vi "Run Test - T90 Plot (SubVI).vi"(8 "error in (no error)":errorcluster, 11 "fileid":string) -> (0 "error out":errorcluster, 3 "Tengent Point":string)   [LabVIEW 2019]
uses:
  Controls/JSON - Report.ctl
  Controls/JSON - GetData.ctl
  <vilib>/httpClient/POSTBuffer.vi
  <userlib>/_OpenG.lib/array/array.llb/Remove Duplicates from 1D Array (String)__ogtk.vi
  <userlib>/_OpenG.lib/array/array.llb/Delete Elements from 1D Array (String)__ogtk.vi
  <vilib>/httpClient/LabVIEWHTTPClient.lvlib
panel:
  out "Array":string[](array[string])
  in  "Generate Report":bool
  in  "Calculate":bool
  in  "Second Point":dbl
  in  "First Point":dbl
  out "Loading":dbl(slide) scale=0.0..100.0
  in  "Test Name":i32(listbox)
  out "Plot":picture
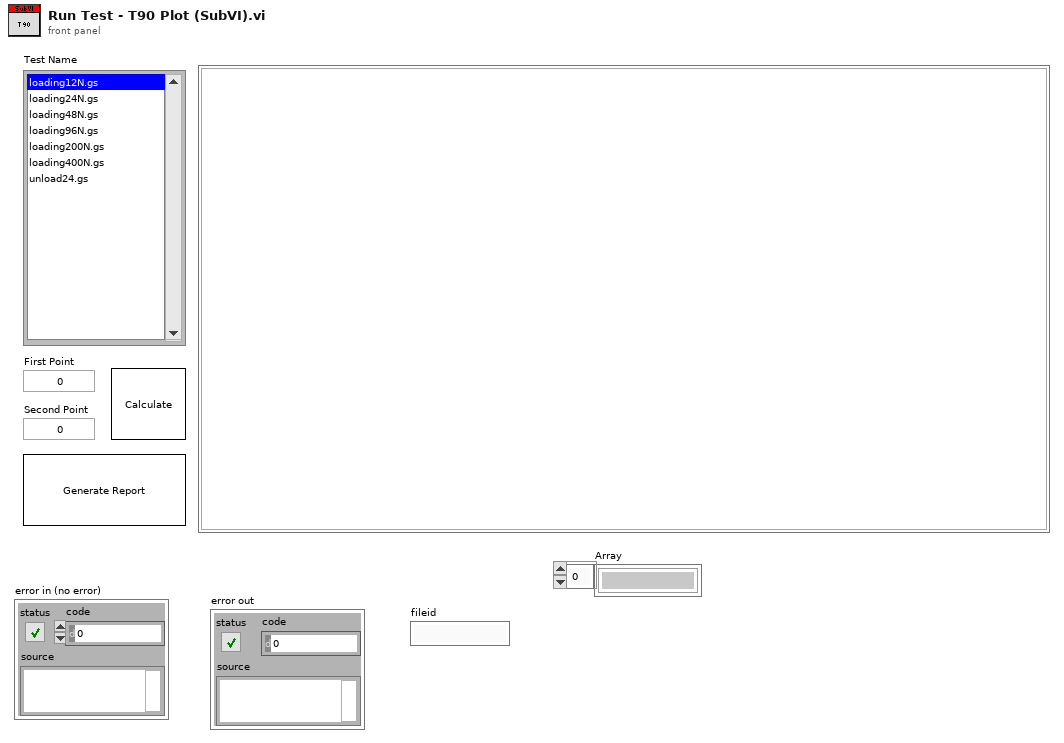
[diagram p1: front panel]
types:
  T1 = typedef "JSON - Report.ctl" = cluster{"status":string, "data":cluster{"testname":string, "testtype":string}[]}
  T2 = typedef "JSON - GetData.ctl" = cluster{"status":string, "data":cluster{"timestamp":string, "elapsetime":string, "testname":string, "testtype":u16, "data":string[]}[]}
  T3 = cluster{"testtype":u16, "testname":string, "fileid":string}
  T4 = cluster{"timestamp":string, "elapsetime":string, "testname":string, "testtype":u16, "data":string[]}[]
  T5 = typedef "imagedata.ctl" = cluster{"image type":i32, "image depth":i32, "image":u8[], "mask":u8[], "colors":u32[], "Rectangle":cluster{"left":i16, "top":i16, "right":i16, "bottom":i16}}
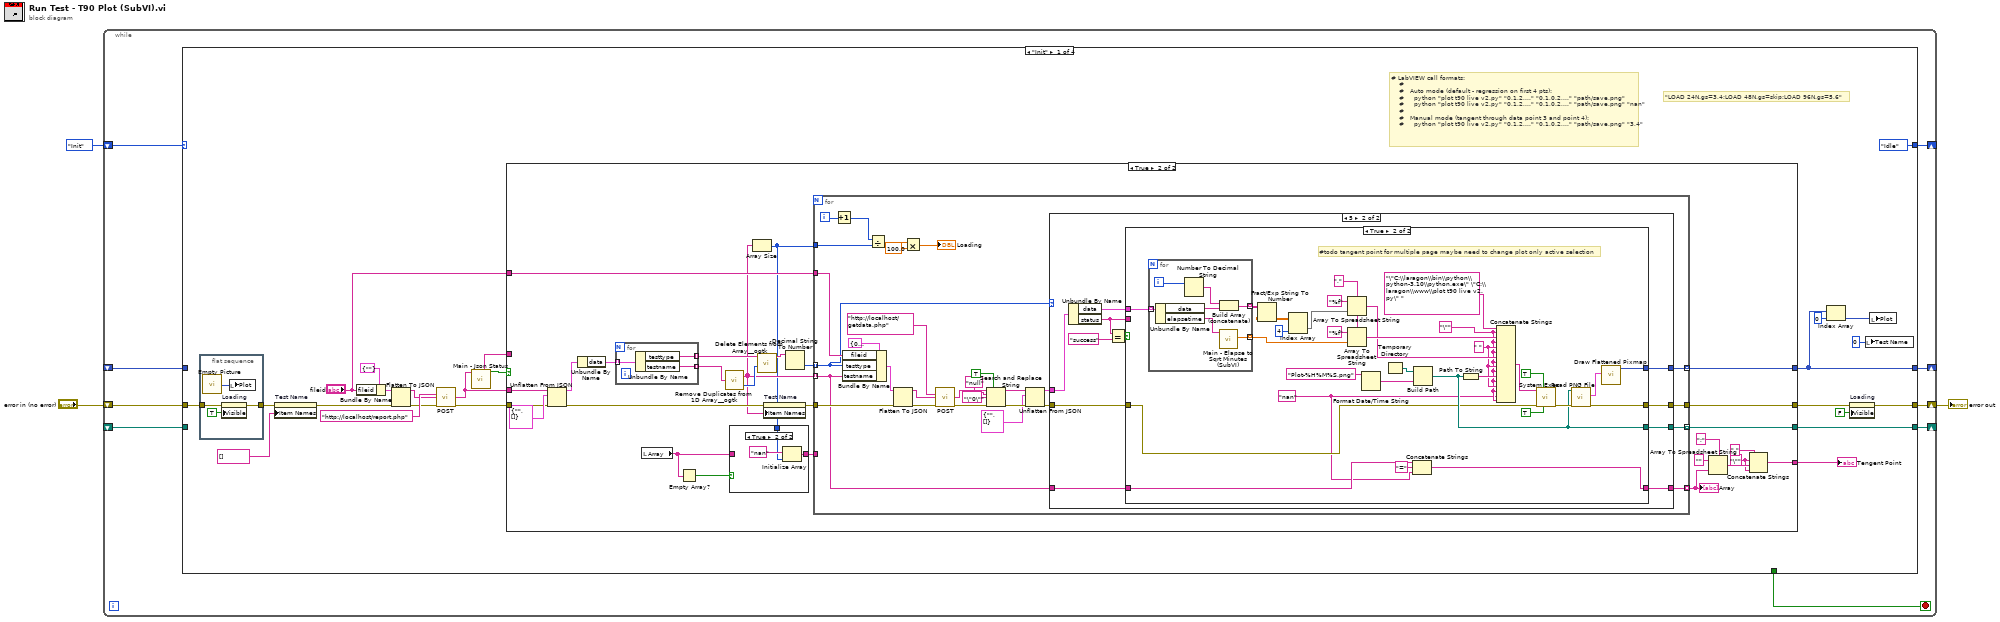
[diagram p0: block diagram]
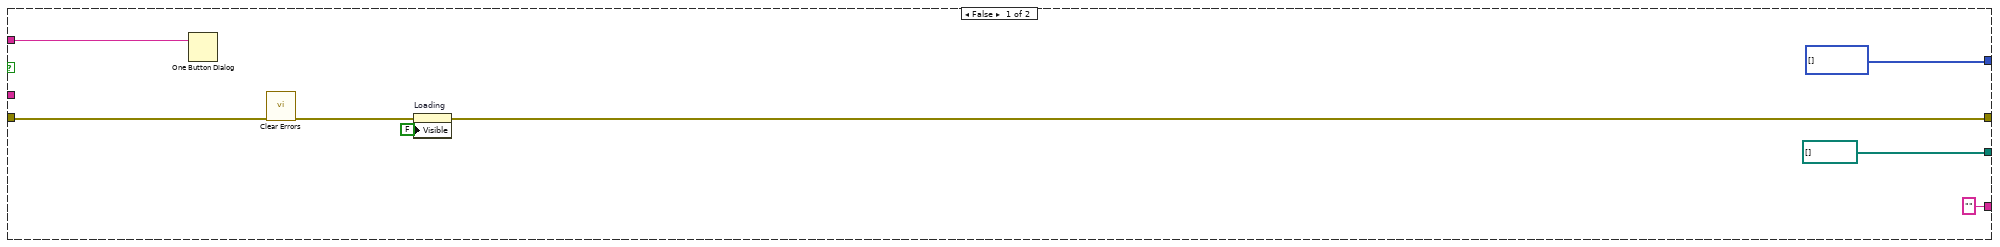
[diagram p2: hidden frame]
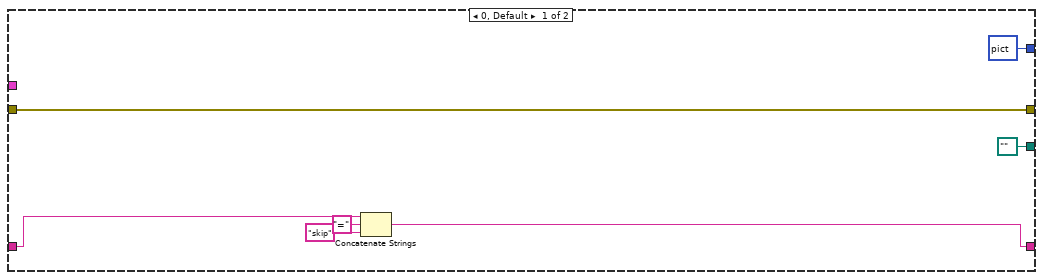
[diagram p4: hidden frame]
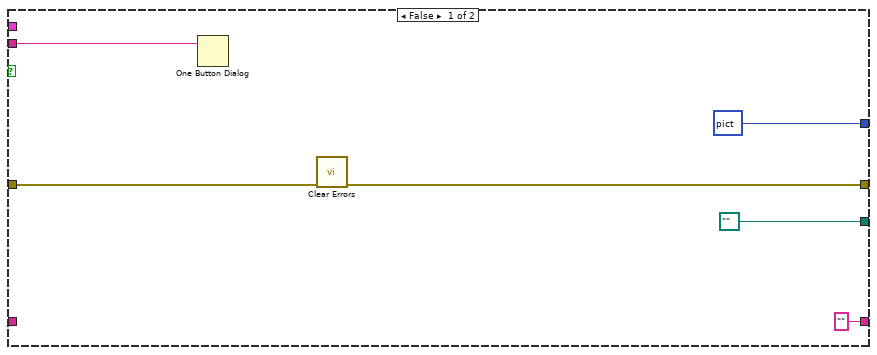
[diagram p5: hidden frame]
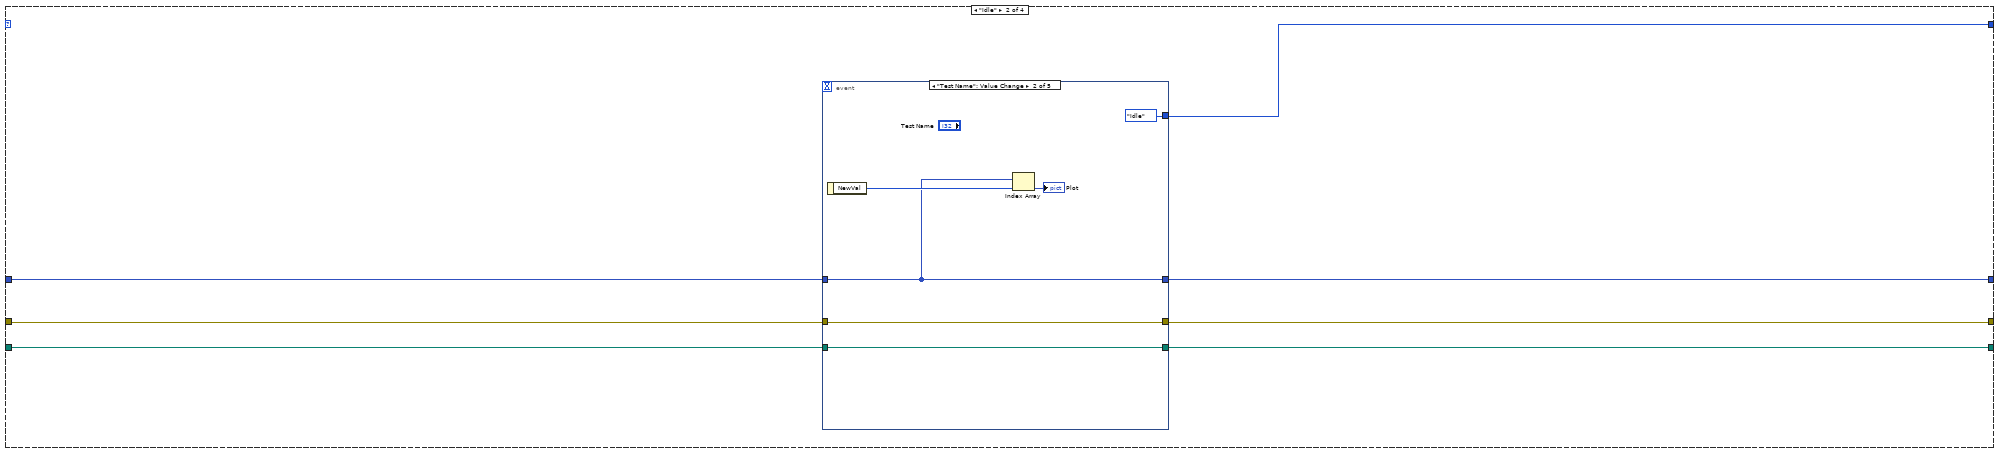
[diagram p6: hidden frame]
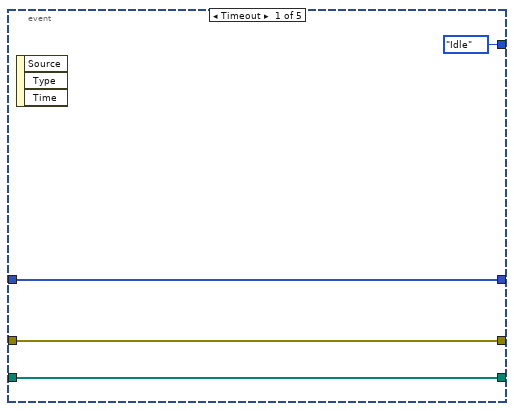
[diagram p7: hidden frame]
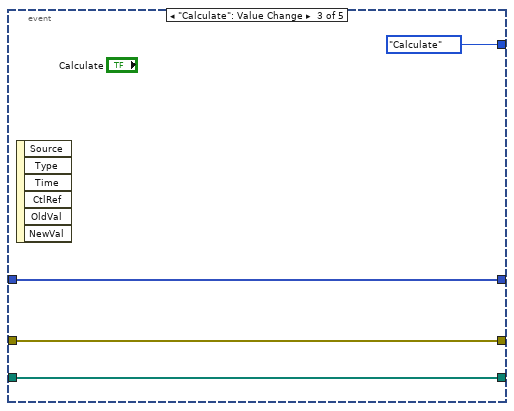
[diagram p8: hidden frame]
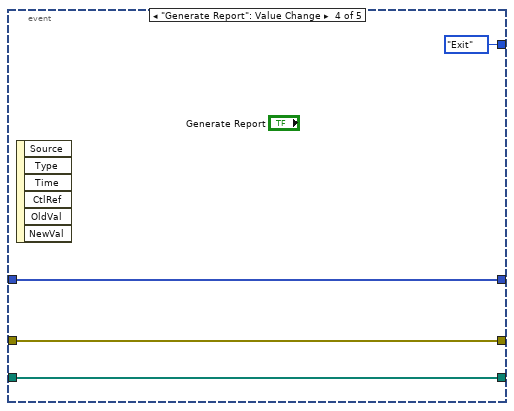
[diagram p9: hidden frame]
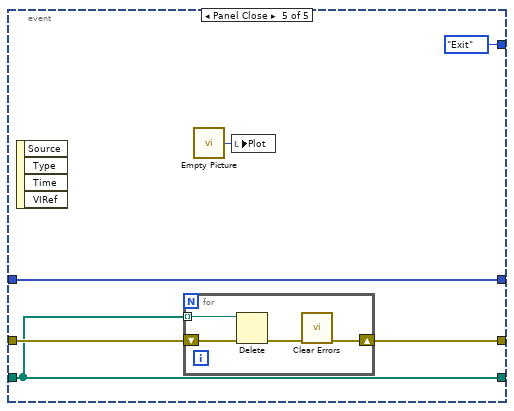
[diagram p10: hidden frame]
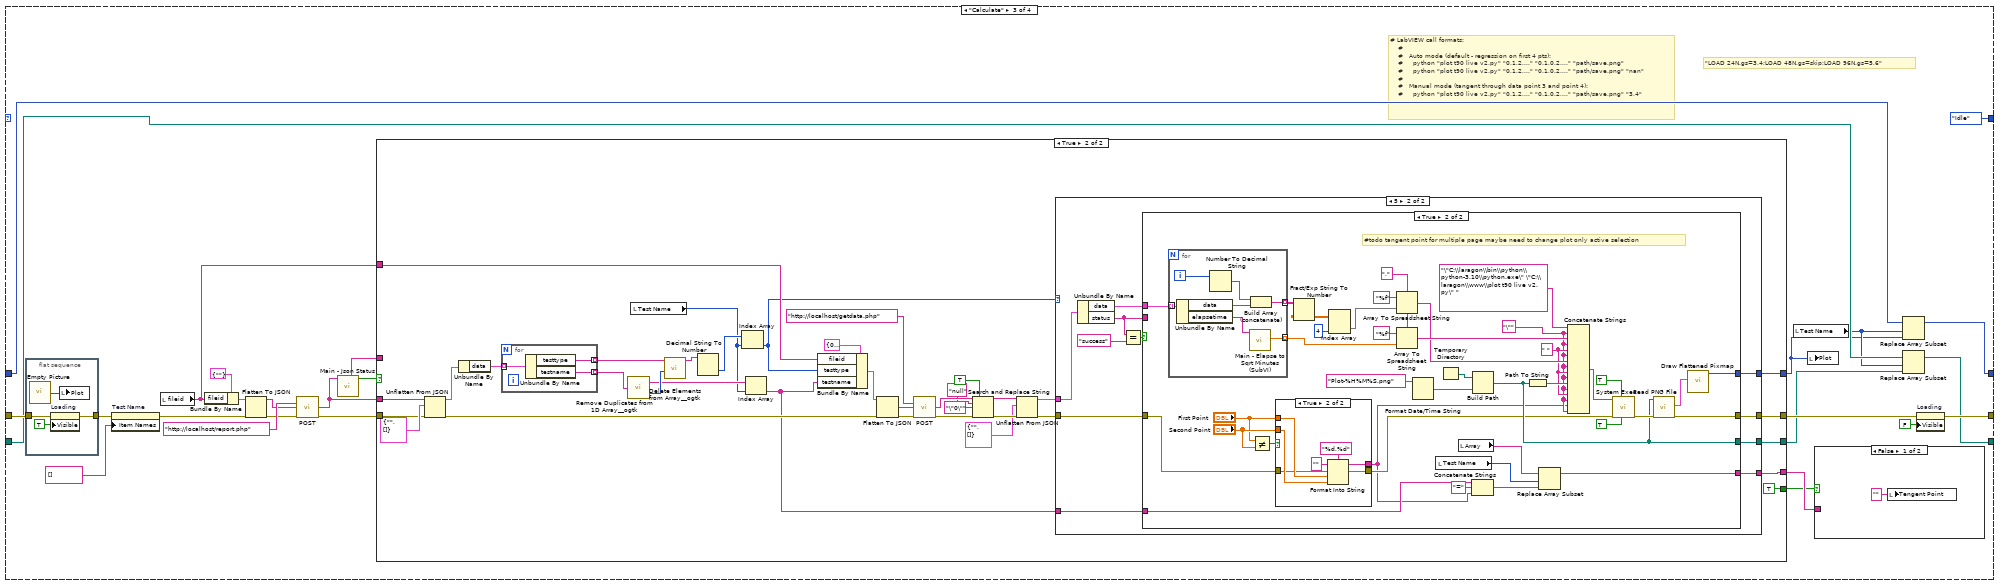
[diagram p11: hidden frame]
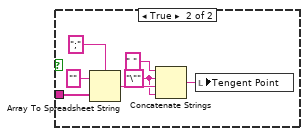
[diagram p12: hidden frame]
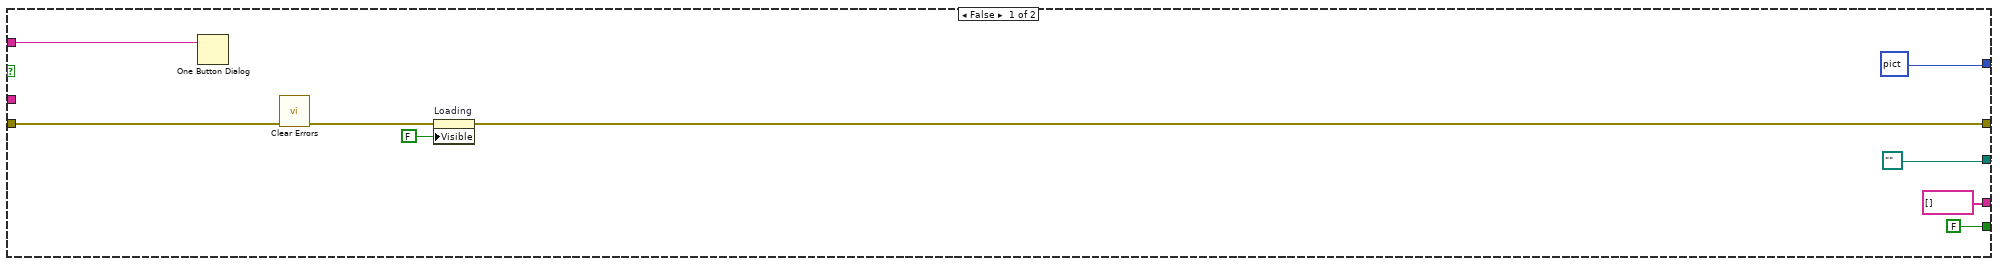
[diagram p13: hidden frame]
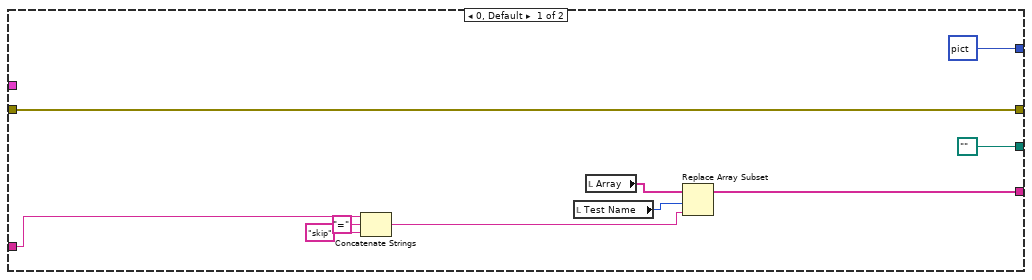
[diagram p14: hidden frame]
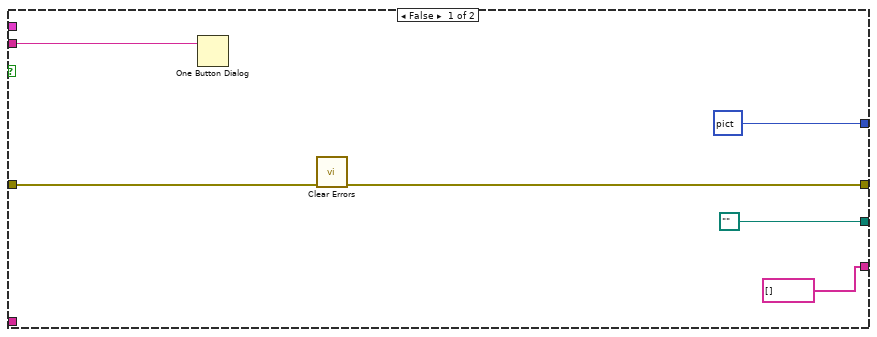
[diagram p15: hidden frame]
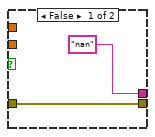
[diagram p16: hidden frame]
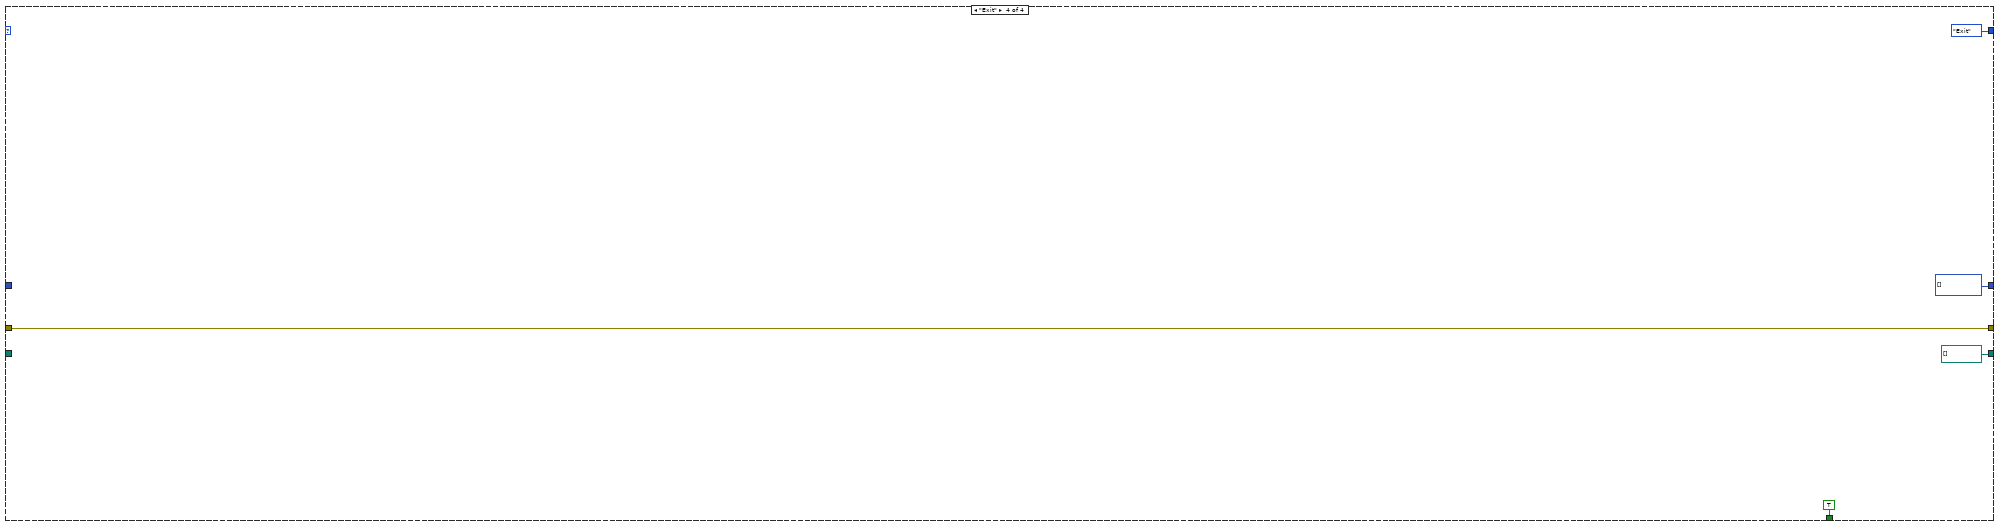
[diagram p17: hidden frame]
diagram:
  n1 = while {
    shift-right: [w11] -> w1
    shift-left: "error in (no error)" -> [w9]
    shift-right: [w7] -> _
    shift-left: enum16{"Init", "Idle", "Calculate", "Exit"}."Init" -> [w8]
    shift-right: [w12] -> _
    shift-left: _ -> [w6]
    shift-right: [w10] -> _
    shift-left: _ -> [w5]
    stop <- w4 stop-if-true
    n2 = case shown="\"Init\"" w8 {
      tunnel: [w26 w177 w216 picture[] []] -> w12
      tunnel: [w22 w178 w226 w379] -> w11
      tunnel: [w17 w176 w215 path[] []] -> w10
      tunnel: w9 -> [w16 w181 w221 w379]
      tunnel: [enum16{"Init", "Idle", "Calculate", "Exit"}."Idle" w175 enum16{"Init", "Idle", "Calculate", "Exit"}."Idle" enum16{"Init", "Idle", "Calculate", "Exit"}."Exit"] -> w7
      tunnel: w6 -> [_ w180 w217 _]
      tunnel: w5 -> [_ w179 w214 _]
      tunnel: [_ _ _ TRUE] -> w4
      frame "Init" {
        # "\"LOAD 24N.gs=3,4;LOAD 48N.gs=skip;LOAD 96N.gs=5,6\""
        # "# LabVIEW call formats:\n    #\n    #   Auto mode (default - regression on first 4 pts):\n    #     python \"plot t90 live v2.py\" \"0,1,2,...\" \"0.1,0.2,...\" \"path/save.png\"\n    #     python \"plot t90 live v2.py\" \"0,1,2,...\" \"0.1,0.2,...\" \"path/save.png\" \"nan\"\n    #\n    #   Manual mode (tangent through data point 3 and point 4):\n    #     python \"plot t90 live v2.py\" \"0,1,2,...\" \"0.1,0.2,...\" \"path/save.png\" \"3,4\""
        n3 = flat-sequence {
          tunnel: [w40] -> w20
          tunnel: w16 -> [w37]
          frame #0 {
            n4 = call "Empty Picture"() -> ("empty picture"=w38:picture)
            n5 = property on="Loading" class="Slide (strict)"(error in=w37, "Visible"=TRUE) -> (error out=w40:errorcluster)  [unwired: 1 in, 1 out]
            n6 = local write "Plot"(w38) -> ()
          }
        }
        n7 = property on="Test Name" class="LstBox (strict)"(error in=w20, "Item Names"=string[] []) -> (error out=w19:errorcluster)  [unwired: 1 in, 1 out]
        n8 = Bundle By Name(cluster=cluster{"fileid":string} {"fileid"=""}, "fileid"="fileid") -> (w35:cluster{"fileid":string})
        n9 = Flatten To JSON(anything=w35, error in (no error)=w19) -> (JSON string=w32:string, 11:w33:errorcluster)  [unwired: 1 in]
        n10 = call-poly <vilib>:"POST.vi"("url"="http://localhost/report.php", "buffer"=w32, "error in (no error)"=w33) -> ("body"=w30:string, "error out"=w31:errorcluster)  [unwired: 9 in, 2 out]
        n11 = call "Main - Json Status.vi"("json"=w30) -> ("Success?"=w29:bool, "message"=w28:string)  [unwired: 9 in]
        n12 = case shown="True" w29 {
          tunnel: w31 -> [w47 w75]
          tunnel: [w43 w65] -> w21
          tunnel: w30 -> [_ w69]
          tunnel: w28 -> [w48 _]
          tunnel: "fileid" -> [_ w68]
          tunnel: [picture[] [] w64] -> w26
          tunnel: [path[] [] w61] -> w17
          tunnel: ["" w49] -> w13
          frame False {
            n13 = One Button Dialog(message=w48) -> ()  [unwired: 1 in, 1 out]
            n14 = call <vilib>:"Clear Errors.vi"("error in (no error)"=w47) -> ("error out"=w44:errorcluster)  [unwired: 5 in, 1 out]
            n15 = property on="Loading" class="Slide (strict)"(error in=w44, "Visible"=FALSE) -> (error out=w43:errorcluster)  [unwired: 1 in, 1 out]
          }
          frame True {
            w51 = "\"" ("string")
            n16 = Unflatten From JSON(JSON string=w69, type and defaults=T1 {"status"="", "data"=[]}, error in (no error)=w75) -> (value=w73:T1, error out=w63:errorcluster)  [unwired: 4 in]
            n17 = Unbundle By Name(w73) -> ("data"=w74:cluster{"testname":string, "testtype":string}[])
            n18 = for {
              tunnel: w74 -> [w174] mode=indexing
              tunnel: [w173] -> w70 mode=indexing
              tunnel: [w172] -> w71 mode=indexing
              n19 = Unbundle By Name(w174) -> ("testtype"=w173:string, "testname"=w172:string)
            }
            n20 = local read "Array"() -> (w56:string[])
            n21 = Empty Array?(array=w56) -> (empty?=w57:bool)
            n22 = call-poly <userlib>:"Remove Duplicates from 1D Array__ogtk.vi"("Input Array"=w71) -> ("Output Array"=w60:string[], "indices of removed elements"=w72:i32[])
            n23 = Array Size(array=w60) -> (size(s)=w59:i32)
            n24 = case shown="True" w57 {
              tunnel: w59 -> [_ w79]
              tunnel: [w77 w78] -> w58
              tunnel: w56 -> [w77 _]
              frame False {
              }
              frame True {
                n25 = Initialize Array("nan" ("element"), w79) -> (w78:string[])
              }
            }
            n26 = call-poly <userlib>:"Delete Elements from Array__ogtk.vi"("indices"=w72, "array"=w70) -> ("array w/ subset deleted"=w67:string[])  [unwired: 8 in, 1 out]
            n27 = property on="Test Name" class="LstBox (strict)"(error in=w63, "Item Names"=w60) -> (error out=w62:errorcluster)  [unwired: 1 in, 1 out]
            n28 = Decimal String To Number(string=w67) -> (number=w66:i32[])  [unwired: 2 in, 1 out]
            n29 = for {
              tunnel: w62 -> [w95]
              tunnel: w68 -> [w94]
              tunnel: w60 -> [w82] mode=indexing
              tunnel: w66 -> [w84] mode=indexing
              tunnel: [w92] -> w65
              tunnel: [w91] -> w64 mode=indexing
              tunnel: w59 -> [w88]
              tunnel: [w85] -> w61 mode=indexing
              tunnel: [w83] -> w55 mode=indexing
              tunnel: w58 -> [_]
              i -> [w90]
              n30 = Increment(x=w90) -> (x+1=w89:i32)
              n31 = Bundle By Name(cluster=T3 {"testtype"=0, "testname"="", "fileid"=""}, "fileid"=w94, "testtype"=w84, "testname"=w82) -> (w109:T3)
              n32 = Divide(x=w89, y=w88) -> (x/y=w87:dbl)
              n33 = Flatten To JSON(anything=w109, error in (no error)=w95) -> (JSON string=w108:string, 11:w98:errorcluster)  [unwired: 1 in]
              n34 = Multiply(x=w87, y=100.0) -> (x*y=→"Loading":dbl)
              n35 = call-poly <vilib>:"POST.vi"("url"="http://localhost/getdata.php", "buffer"=w108, "error in (no error)"=w98) -> ("body"=w105:string, "error out"=w97:errorcluster)  [unwired: 9 in, 2 out]
              n36 = Search and Replace String(replace all?=TRUE ("replace all? (F)"), input string=w105, search string="null", replace string="\"0\"" ("replace string (\"\")"), error in=w97) -> (result string=w104:string, error out=w106:errorcluster)  [unwired: 3 in, 2 out]
              n37 = Unflatten From JSON(JSON string=w104, type and defaults=T2 {"status"="", "data"=[]}, error in (no error)=w106) -> (value=w107:T2, error out=w93:errorcluster)  [unwired: 4 in]
              n38 = case shown="5" w84 {
                tunnel: w107 -> [_ w127]
                tunnel: w93 -> [w116 w123]
                tunnel: [w116 w122] -> w92
                tunnel: [picture data[5B] ("new picture") w121] -> w91
                tunnel: [path "" ("appended path") w119] -> w85
                tunnel: w82 -> [w112 w118]
                tunnel: [w110 w117] -> w83
                frame 0, Default {
                  n39 = Concatenate Strings(w112, "=" ("string"), "skip" ("string")) -> (w110:string)
                }
                frame 5 {
                  n40 = Unbundle By Name(w127) -> ("data"=w125:T4, "status"=w120:string)
                  n41 = Equal?(x=w120, y="success") -> (x = y?=w124:bool)
                  n42 = case shown="True" w124 {
                    tunnel: w125 -> [_ w163]
                    tunnel: w123 -> [w132 w140]
                    tunnel: [w130 w143] -> w122
                    tunnel: [picture data[5B] ("new picture") w142] -> w121
                    tunnel: w120 -> [w131 _]
                    tunnel: [path "" ("appended path") w141] -> w119
                    tunnel: w118 -> [_ w139]
                    tunnel: ["" ("Array") w134] -> w117
                    frame False {
                      n43 = One Button Dialog(message=w131) -> ()  [unwired: 1 in, 1 out]
                      n44 = call <vilib>:"Clear Errors.vi"("error in (no error)"=w132) -> ("error out"=w130:errorcluster)  [unwired: 5 in, 1 out]
                    }
                    frame True {
                      w135 = "nan"
                      w137 = " " ("string")
                      w136 = "\"" ("string")
                      w156 = "," ("delimiter (Tab)")
                      # "#todo tangent point for multiple page maybe need to change plot only active selection"
                      n45 = for {
                        tunnel: w163 -> [w171] mode=indexing
                        tunnel: [w169] -> w164 mode=indexing
                        tunnel: [w165] -> w157 mode=indexing
                        i -> [w167]
                        n46 = Unbundle By Name(w171) -> ("data"=w170:string[], "elapsetime"=w166:string)
                        n47 = Number To Decimal String(number=w167) -> (decimal integer string=w168:string)  [unwired: 1 in]
                        n48 = call "Main - Elapse to Sqrt Minutes (SubVI).vi"("Elapse"=w166) -> ("sqrt (Minute)"=w165:dbl)  [unwired: 9 in, 1 out]
                        n49 = Build Array (concatenate)(w168, w170) -> (w169:string[])
                      }
                      n50 = Fract/Exp String To Number(string=w164) -> (number=w160:dbl[][])  [unwired: 3 in, 1 out]
                      n51 = Index Array(array=w160, index (col)=4 ("disabled index (col)")) -> (element=w159:dbl[])  [unwired: 1 in]
                      n52 = Array To Spreadsheet String(delimiter (Tab)=w156, array=w159, 3:"%f" ("format string")) -> (spreadsheet string=w149:string)
                      n53 = Array To Spreadsheet String(delimiter (Tab)=w156, array=w157, 3:"%f" ("format string")) -> (spreadsheet string=w150:string)
                      n54 = Format Date/Time String(time format string (%c)="Plot-%H%M%S.png") -> (date/time string=w152:string)  [unwired: 2 in]
                      n55 = Temporary Directory() -> (w154:path)
                      n56 = Concatenate Strings(w139, "=" ("string"), w135) -> (w134:string)
                      n57 = Build Path(base path=w154, name or relative path=w152) -> (appended path=w141:path)
                      n58 = Path To String(path=w141) -> (string=w151:string)
                      n59 = Concatenate Strings("\"C:\\laragon\\bin\\python\\python-3.10\\python.exe\" \"C:\\laragon\\www\\plot t90 live v2.py\" " ("y"), w136, w150, w136, w137, w136, w149, w136, w137, w136, w151, w136, w137, w136, w135, w136) -> (w146:string)
                      n60 = call <vilib>:"System Exec.vi"("run minimized? (F)"=TRUE, "wait until completion? (T)"=TRUE, "error in (no error)"=w140, "command line"=w146) -> ("error out"=w144:errorcluster)  [unwired: 4 in, 3 out]
                      n61 = call <vilib>:"Read PNG File.vi"("error in (no error)"=w144, "path to PNG file"=w141) -> ("error out"=w143:errorcluster, "image data"=w145:T5)  [unwired: 7 in, 1 out]
                      n62 = call <vilib>:"Draw Flattened Pixmap.vi"("image data"=w145) -> ("new picture"=w142:picture)  [unwired: 8 in]
                    }
                  }
                }
              }
            }
            "Array" <- w55
            n63 = Array To Spreadsheet String(delimiter (Tab)=";", array=w55, 3:"" ("format string")) -> (spreadsheet string=w52:string)
            n64 = Concatenate Strings(" " ("string"), w51, w52, w51) -> (w49:string)
          }
        }
        "Tengent Point" <- w13
        n65 = Index Array(array=w26, index=0) -> (element=w25:picture)
        n66 = property on="Loading" class="Slide (strict)"(error in=w21, "Visible"=FALSE) -> (error out=w22:errorcluster)  [unwired: 1 in, 1 out]
        n67 = local write "Test Name"(0 ("Test Name")) -> ()
        n68 = local write "Plot"(w25) -> ()
      }
      frame "Idle" {
        n69 = event shown="[1] \"Test Name\": Value Change" {
          selector: _ -> [_ _ _ _ _]
          dyn-events: _ -> [_ _ _ _ _]
          timeout: _ -> [_ _ _ _ _]
          tunnel: w180 -> [w184 w188 w194 w197 w202]
          tunnel: w181 -> [w185 w189 w195 w199 w203]
          tunnel: [w185 w189 w195 w199 w204] -> w178
          tunnel: w179 -> [w183 w187 w193 w196 w201]
          tunnel: [w184 w188 w194 w197 w202] -> w177
          tunnel: [w183 w187 w193 w196 w201] -> w176
          tunnel: [enum16{"Init", "Idle", "Calculate", "Exit"}."Idle" enum16{"Init", "Idle", "Calculate", "Exit"}."Idle" enum16{"Init", "Idle", "Calculate", "Exit"}."Calculate" enum16{"Init", "Idle", "Calculate", "Exit"}."Exit" enum16{"Init", "Idle", "Calculate", "Exit"}."Exit"] -> w175
          event Timeout {
            n70 = event-data() -> ()  [unwired: 1 in, 3 out]
          }
          event "Test Name": Value Change {
            n71 = event-data() -> ("NewVal"=w191:i32)  [unwired: 1 in]
            n72 = Index Array(array=w188, index=w191) -> (element=→"Plot":picture)
          }
          event "Calculate": Value Change {
            n73 = event-data() -> ()  [unwired: 1 in, 6 out]
          }
          event "Generate Report": Value Change {
            n74 = event-data() -> ()  [unwired: 1 in, 6 out]
          }
          event Panel Close {
            n75 = event-data() -> ()  [unwired: 1 in, 4 out]
            n76 = for {
              tunnel: w201 -> [w207] mode=indexing
              shift-right: [w206] -> w204
              shift-left: w203 -> [w208]
              n77 = Delete(path (use dialog)=w207, error in=w208) -> (error out=w209:errorcluster)  [unwired: 3 in, 2 out]
              n78 = call <vilib>:"Clear Errors.vi"("error in (no error)"=w209) -> ("error out"=w206:errorcluster)  [unwired: 5 in, 1 out]
            }
            n79 = call "Empty Picture"() -> ("empty picture"=w205:picture)
            n80 = local write "Plot"(w205) -> ()
          }
        }
      }
      frame "Calculate" {
        # "\"LOAD 24N.gs=3,4;LOAD 48N.gs=skip;LOAD 96N.gs=5,6\""
        # "# LabVIEW call formats:\n    #\n    #   Auto mode (default - regression on first 4 pts):\n    #     python \"plot t90 live v2.py\" \"0,1,2,...\" \"0.1,0.2,...\" \"path/save.png\"\n    #     python \"plot t90 live v2.py\" \"0,1,2,...\" \"0.1,0.2,...\" \"path/save.png\" \"nan\"\n    #\n    #   Manual mode (tangent through data point 3 and point 4):\n    #     python \"plot t90 live v2.py\" \"0,1,2,...\" \"0.1,0.2,...\" \"path/save.png\" \"3,4\""
        n81 = flat-sequence {
          tunnel: [w248] -> w224
          tunnel: w221 -> [w245]
          frame #0 {
            n82 = call "Empty Picture"() -> ("empty picture"=w246:picture)
            n83 = property on="Loading" class="Slide (strict)"(error in=w245, "Visible"=TRUE) -> (error out=w248:errorcluster)  [unwired: 1 in, 1 out]
            n84 = local write "Plot"(w246) -> ()
          }
        }
        n85 = property on="Test Name" class="LstBox (strict)"(error in=w224, "Item Names"=string[] []) -> (error out=w223:errorcluster)  [unwired: 1 in, 1 out]
        n86 = local read "fileid"() -> (w219:string)
        n87 = Bundle By Name(cluster=cluster{"fileid":string} {"fileid"=""}, "fileid"=w219) -> (w235:cluster{"fileid":string})
        n88 = Flatten To JSON(anything=w235, error in (no error)=w223) -> (JSON string=w232:string, 11:w233:errorcluster)  [unwired: 1 in]
        n89 = call-poly <vilib>:"POST.vi"("url"="http://localhost/report.php", "buffer"=w232, "error in (no error)"=w233) -> ("body"=w230:string, "error out"=w231:errorcluster)  [unwired: 9 in, 2 out]
        n90 = call "Main - Json Status.vi"("json"=w230) -> ("Success?"=w229:bool, "message"=w228:string)  [unwired: 9 in]
        n91 = case shown="True" w229 {
          tunnel: w231 -> [w256 w292]
          tunnel: [w253 w283] -> w225
          tunnel: w230 -> [_ w286]
          tunnel: w228 -> [w257 _]
          tunnel: w219 -> [_ w285]
          tunnel: [picture data[5B] ("new picture") w282] -> w211
          tunnel: [path "" ("appended path") w281] -> w213
          tunnel: [string[] [] ("Array") w259] -> w218
          tunnel: [FALSE TRUE] -> w210
          frame False {
            n92 = One Button Dialog(message=w257) -> ()  [unwired: 1 in, 1 out]
            n93 = call <vilib>:"Clear Errors.vi"("error in (no error)"=w256) -> ("error out"=w254:errorcluster)  [unwired: 5 in, 1 out]
            n94 = property on="Loading" class="Slide (strict)"(error in=w254, "Visible"=FALSE) -> (error out=w253:errorcluster)  [unwired: 1 in, 1 out]
          }
          frame True {
            n95 = Unflatten From JSON(JSON string=w286, type and defaults=T1 {"status"="", "data"=[]}, error in (no error)=w292) -> (value=w290:T1, error out=w265:errorcluster)  [unwired: 4 in]
            n96 = Unbundle By Name(w290) -> ("data"=w291:cluster{"testname":string, "testtype":string}[])
            n97 = for {
              tunnel: w291 -> [w377] mode=indexing
              tunnel: [w376] -> w287 mode=indexing
              tunnel: [w375] -> w288 mode=indexing
              n98 = Unbundle By Name(w377) -> ("testtype"=w376:string, "testname"=w375:string)
            }
            n99 = call-poly <userlib>:"Remove Duplicates from 1D Array__ogtk.vi"("Input Array"=w288) -> ("Output Array"=w263:string[], "indices of removed elements"=w289:i32[])
            n100 = local read "Test Name"() -> (w262:i32)
            n101 = call-poly <userlib>:"Delete Elements from Array__ogtk.vi"("indices"=w289, "array"=w287) -> ("array w/ subset deleted"=w284:string[])  [unwired: 8 in, 1 out]
            n102 = Decimal String To Number(string=w284) -> (number=w264:i32[])  [unwired: 2 in, 1 out]
            n103 = Index Array(array=w264, index=w262) -> (element=w260:i32)
            n104 = Index Array(array=w263, index=w262) -> (element=w261:string)
            n105 = Bundle By Name(cluster=T3 {"testtype"=0, "testname"="", "fileid"=""}, "fileid"=w285, "testtype"=w260, "testname"=w261) -> (w280:T3)
            n106 = Flatten To JSON(anything=w280, error in (no error)=w265) -> (JSON string=w279:string, 11:w269:errorcluster)  [unwired: 1 in]
            n107 = call-poly <vilib>:"POST.vi"("url"="http://localhost/getdata.php", "buffer"=w279, "error in (no error)"=w269) -> ("body"=w276:string, "error out"=w268:errorcluster)  [unwired: 9 in, 2 out]
            n108 = Search and Replace String(replace all?=TRUE ("replace all? (F)"), input string=w276, search string="null", replace string="\"0\"" ("replace string (\"\")"), error in=w268) -> (result string=w275:string, error out=w277:errorcluster)  [unwired: 3 in, 2 out]
            n109 = Unflatten From JSON(JSON string=w275, type and defaults=T2 {"status"="", "data"=[]}, error in (no error)=w277) -> (value=w278:T2, error out=w266:errorcluster)  [unwired: 4 in]
            n110 = case shown="5" w260 {
              tunnel: w278 -> [_ w314]
              tunnel: w266 -> [w303 w310]
              tunnel: [w303 w309] -> w283
              tunnel: [picture data[5B] ("new picture") w308] -> w282
              tunnel: [path "" ("appended path") w306] -> w281
              tunnel: w261 -> [w297 w305]
              tunnel: [w294 w304] -> w259
              frame 0, Default {
                n111 = Concatenate Strings(w297, "=" ("string"), "skip" ("string")) -> (w299:string)
                n112 = local read "Test Name"() -> (w300:i32)
                n113 = local read "Array"() -> (w295:string[])
                n114 = Replace Array Subset(array=w295, new element=w299, index=w300) -> (w294:string[])
              }
              frame 5 {
                n115 = Unbundle By Name(w314) -> ("data"=w312:T4, "status"=w307:string)
                n116 = Equal?(x=w307, y="success") -> (x = y?=w311:bool)
                n117 = case shown="True" w311 {
                  tunnel: w312 -> [_ w357]
                  tunnel: w310 -> [w319 w331]
                  tunnel: [w317 w337] -> w309
                  tunnel: [picture data[5B] ("new picture") w336] -> w308
                  tunnel: w307 -> [w318 _]
                  tunnel: [path "" ("appended path") w335] -> w306
                  tunnel: w305 -> [_ w329]
                  tunnel: [string[] [] ("Array") w321] -> w304
                  frame False {
                    n118 = One Button Dialog(message=w318) -> ()  [unwired: 1 in, 1 out]
                    n119 = call <vilib>:"Clear Errors.vi"("error in (no error)"=w319) -> ("error out"=w317:errorcluster)  [unwired: 5 in, 1 out]
                  }
                  frame True {
                    w327 = " " ("string")
                    w326 = "\"" ("string")
                    w350 = "," ("delimiter (Tab)")
                    # "#todo tangent point for multiple page maybe need to change plot only active selection"
                    n120 = for {
                      tunnel: w357 -> [w374] mode=indexing
                      tunnel: [w372] -> w358 mode=indexing
                      tunnel: [w368] -> w351 mode=indexing
                      i -> [w370]
                      n121 = Unbundle By Name(w374) -> ("data"=w373:string[], "elapsetime"=w369:string)
                      n122 = Number To Decimal String(number=w370) -> (decimal integer string=w371:string)  [unwired: 1 in]
                      n123 = call "Main - Elapse to Sqrt Minutes (SubVI).vi"("Elapse"=w369) -> ("sqrt (Minute)"=w368:dbl)  [unwired: 9 in, 1 out]
                      n124 = Build Array (concatenate)(w371, w373) -> (w372:string[])
                    }
                    n125 = Not Equal?(x="First Point", y="Second Point") -> (x != y?=w334:bool)
                    n126 = case shown="True" w334 {
                      tunnel: ["nan" w365] -> w325
                      tunnel: "First Point" -> [_ w364]
                      tunnel: "Second Point" -> [_ w363]
                      tunnel: w331 -> [w359 w362]
                      tunnel: [w359 w361] -> w330
                      frame False {
                      }
                      frame True {
                        n127 = Format Into String(format string="%d,%d", initial string="", error in=w362, w364, w363) -> (resulting string=w365:string, error out=w361:errorcluster)
                      }
                    }
                    n128 = Fract/Exp String To Number(string=w358) -> (number=w354:dbl[][])  [unwired: 3 in, 1 out]
                    n129 = Index Array(array=w354, index (col)=4 ("disabled index (col)")) -> (element=w353:dbl[])  [unwired: 1 in]
                    n130 = Array To Spreadsheet String(delimiter (Tab)=w350, array=w353, 3:"%f" ("format string")) -> (spreadsheet string=w343:string)
                    n131 = Array To Spreadsheet String(delimiter (Tab)=w350, array=w351, 3:"%f" ("format string")) -> (spreadsheet string=w344:string)
                    n132 = Format Date/Time String(time format string (%c)="Plot-%H%M%S.png") -> (date/time string=w346:string)  [unwired: 2 in]
                    n133 = local read "Test Name"() -> (w322:i32)
                    n134 = Temporary Directory() -> (w348:path)
                    n135 = local read "Array"() -> (w324:string[])
                    n136 = Concatenate Strings(w329, "=" ("string"), w325) -> (w323:string)
                    n137 = Build Path(base path=w348, name or relative path=w346) -> (appended path=w335:path)
                    n138 = Path To String(path=w335) -> (string=w345:string)
                    n139 = Replace Array Subset(array=w324, new element=w323, index=w322) -> (w321:string[])
                    n140 = Concatenate Strings("\"C:\\laragon\\bin\\python\\python-3.10\\python.exe\" \"C:\\laragon\\www\\plot t90 live v2.py\" " ("y"), w326, w344, w326, w327, w326, w343, w326, w327, w326, w345, w326, w327, w326, w325, w326) -> (w340:string)
                    n141 = call <vilib>:"System Exec.vi"("run minimized? (F)"=TRUE, "wait until completion? (T)"=TRUE, "error in (no error)"=w330, "command line"=w340) -> ("error out"=w338:errorcluster)  [unwired: 4 in, 3 out]
                    n142 = call <vilib>:"Read PNG File.vi"("error in (no error)"=w338, "path to PNG file"=w335) -> ("error out"=w337:errorcluster, "image data"=w339:T5)  [unwired: 7 in, 1 out]
                    n143 = call <vilib>:"Draw Flattened Pixmap.vi"("image data"=w339) -> ("new picture"=w336:picture)  [unwired: 8 in]
                  }
                }
              }
            }
          }
        }
        n144 = local read "Test Name"() -> (w212:i32)
        n145 = local write "Plot"(w211) -> ()
        n146 = case shown="False" w210 {
          tunnel: w218 -> [_ w239]
          frame False {
            n147 = local write "Tengent Point"("" ("Tengent Point")) -> ()
          }
          frame True {
            w242 = "\"" ("string")
            n148 = Array To Spreadsheet String(delimiter (Tab)=";", array=w239, 3:"" ("format string")) -> (spreadsheet string=w244:string)
            n149 = Concatenate Strings(" " ("string"), w242, w244, w242) -> (w238:string)
            n150 = local write "Tengent Point"(w238) -> ()
          }
        }
        n151 = Replace Array Subset(array=w217, new element=w211, index=w212) -> (w216:picture[])
        n152 = Replace Array Subset(array=w214, new element=w213, index=w212) -> (w215:path[])
        n153 = property on="Loading" class="Slide (strict)"(error in=w225, "Visible"=FALSE) -> (error out=w226:errorcluster)  [unwired: 1 in, 1 out]
      }
      frame "Exit" {
      }
    }
  }
  "error out" <- w1
